vi "Create Fast Draw Object.vi"(6 "Actual Transform In":T1, 8 "error in (no error)":errorcluster, 9 "Multiplot Representation In":T3, 10 "3D Quiver.lvclass in":refnum<class "3D Quiver.lvclass">, 11 "Plot Object In":refnum<vi>) -> (0 "error out":errorcluster, 1 "Multiplot Representation Out":T3, 2 "3D Quiver.lvclass out":refnum<class "3D Quiver.lvclass">, 3 "Plot Object Out":refnum<vi>, 4 "Actual Transform Out":T1)   [LabVIEW 2020, in "3D Quiver.lvclass"]
uses:
  <vilib>/Math Plots/3D Math Plots/3D Quiver/3D Quiver/3D Quiver.lvclass
  <vilib>/Math Plots/3D Math Plots/3D Plot/3D Plot/Typedef/Multiplot Representation.ctl
  <vilib>/Math Plots/3D Math Plots/3D Plot/3D Plot/Typedef/Plot Representation.ctl
  <vilib>/Math Plots/3D Math Plots/3D Plot/3D Plot/Typedef/Range Clusters.ctl
  <vilib>/Math Plots/3D Math Plots/3D Plot/3D Plot/Typedef/Mesh Data.ctl
  <vilib>/Math Plots/3D Math Plots/3D Plot/3D Plot/Typedef/Actual Transform.ctl
  <vilib>/Math Plots/3D Math Plots/3D Quiver/3D Quiver/3D Quiver.lvclass/3D Quiver.ctl
  <vilib>/Math Plots/3D Math Plots/3D Plot/3D Plot/3D Plot.lvclass
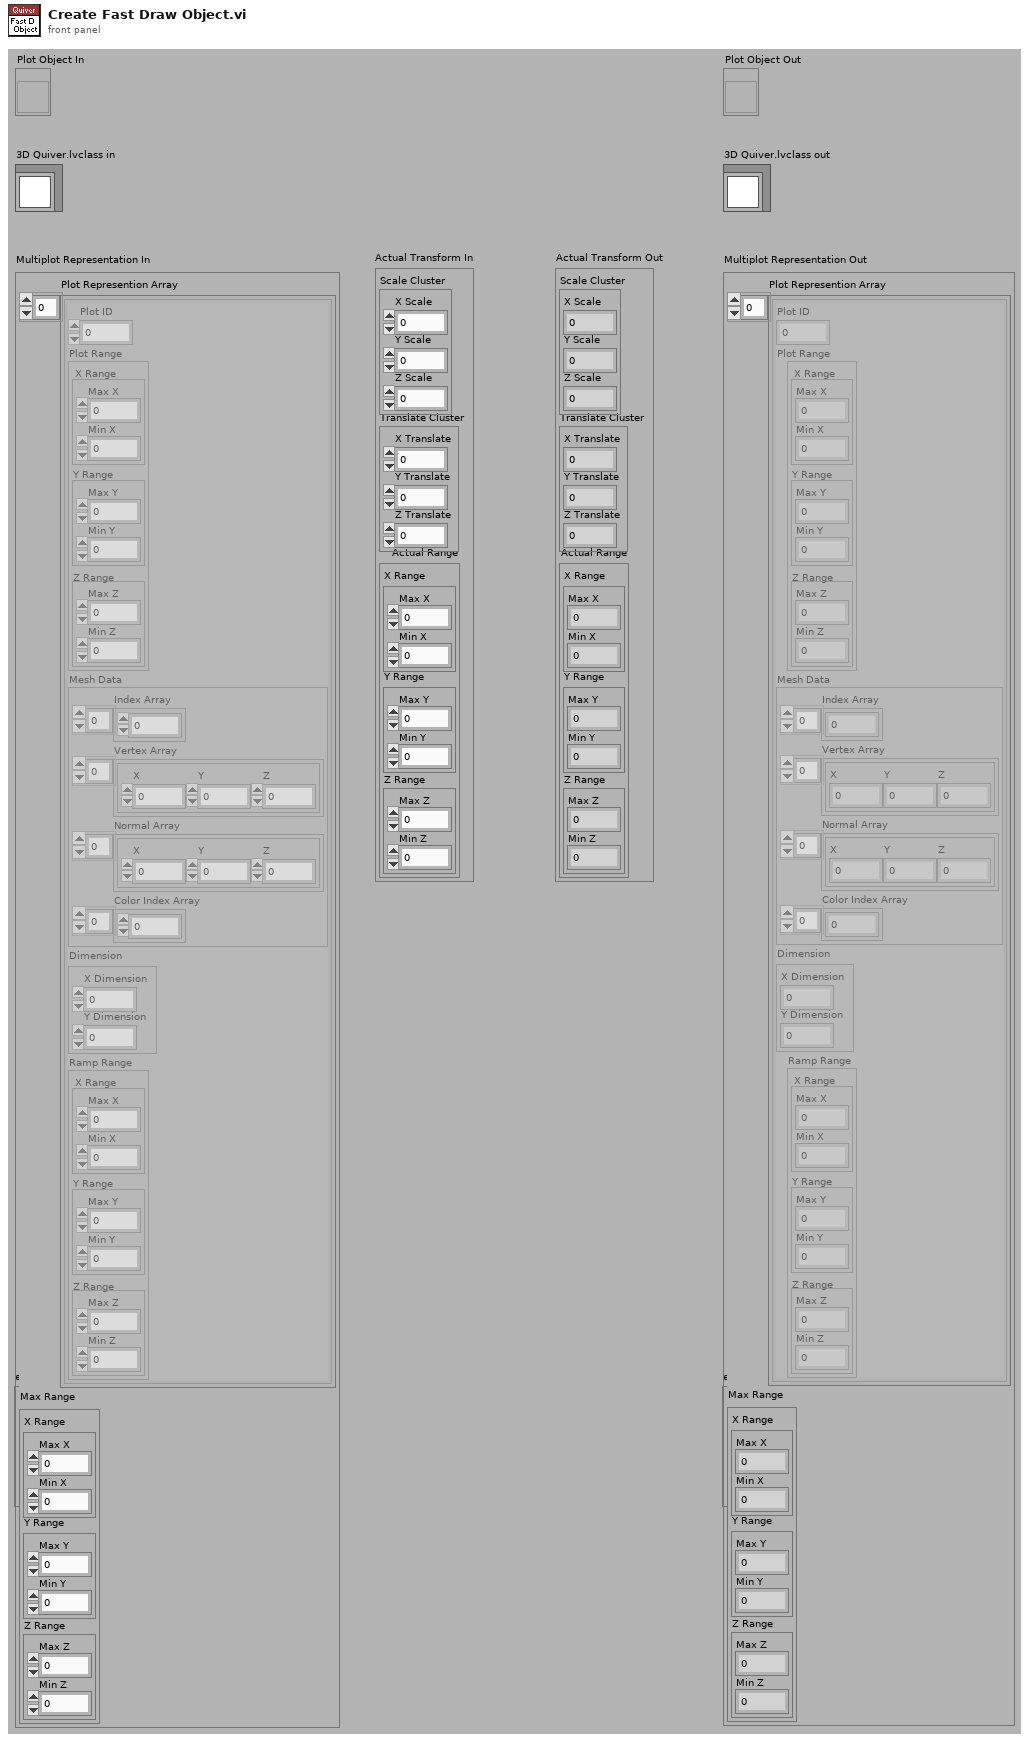
[diagram p1: front panel]
types:
  T1 = typedef "3D Plot.lvclass/Actual Transform.ctl" = cluster{"Scale Cluster":cluster{"X Scale":sgl, "Y Scale":sgl, "Z Scale":sgl}, "Translate Cluster":cluster{"X Translate":sgl, "Y Translate":sgl, "Z Translate":sgl}, "Actual Range":T2}
  T2 = typedef "3D Plot.lvclass/Range Clusters.ctl" = cluster{"X Range":cluster{"Max X":sgl, "Min X":sgl}, "Y Range":cluster{"Max Y":sgl, "Min Y":sgl}, "Z Range":cluster{"Max Z":sgl, "Min Z":sgl}}
  T3 = typedef "3D Plot.lvclass/Multiplot Representation.ctl" = cluster{"Plot Represention Array":T4[], "Max Range":T2}
  T4 = typedef "3D Plot.lvclass/Plot Representation.ctl" = cluster{"Plot ID":i32, "Plot Range":T2, "Mesh Data":T5, "Dimension":cluster{"X Dimension":i32, "Y Dimension":i32}, "Ramp Range":T2}
  T5 = typedef "3D Plot.lvclass/Mesh Data.ctl" = cluster{"Index Array":u32[], "Vertex Array":cluster{"X":sgl, "Y":sgl, "Z":sgl}[], "Normal Array":cluster{"X":sgl, "Y":sgl, "Z":sgl}[], "Color Index Array":i32[]}
  T6 = typedef "3D Quiver.lvclass/3D Quiver Property Array.ctl" = T7[]
  T7 = typedef "3D Quiver.lvclass/3D Quiver Property.ctl" = cluster{"General Property":cluster{"Plot Name":string, "Coordinate System":enum16{"Cartesian", "Cylindrical", "Spherical"}, "Opacity":sgl}, "Projection Property":cluster{"Draw XY":bool, "Draw YZ":bool, "Draw XZ":bool}, "Plot Property":cluster{"Line Style":T8, "Line Width":sgl, "Line Color":u32, "Antialiasing":bool, "Color Ramp Cluster":T9}, "Quiver Property":cluster{"Quvier Mode":enum16{"Quiver", "Quiver with surface"}, "Quiver Size":sgl, "Quiver Length":sgl}}
  T8 = typedef "3D Plot.lvclass/Line Type.ctl" = enum16{"None", "Solid", "Dash", "Dot", "Dash Dot"}
  T9 = typedef "3D Plot.lvclass/Color Ramp Cluster.ctl" = cluster{"Color Ramp Style":enum16{"None", "Shaded", "Color spectrum", "Grey scale", "Custom"}, "Color Ramp Array":u32[], "Color Ramp Index":i32[], "Interpolate?":bool, "Logarithm?":bool}
  T10 = enum16{"Points", "Lines", "Line Strip", "Line Loop", "Triangles", "Triangle Strip", "Triangle Fan", "Quads", "Quad Strip", "Polygon"}
  T11 = cluster{"Draw XY":bool, "Draw YZ":bool, "Draw XZ":bool}
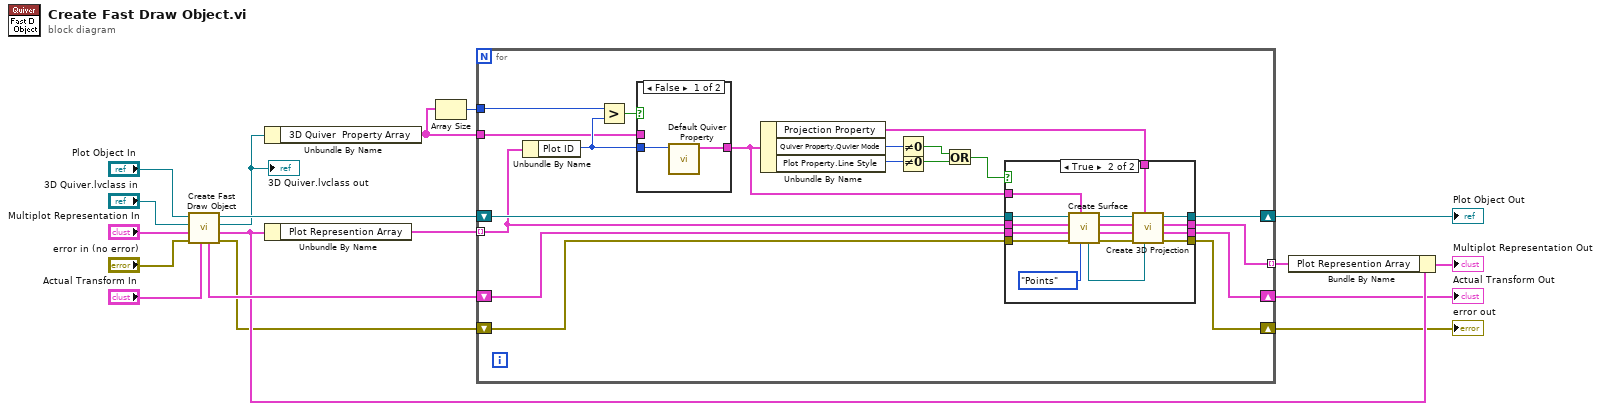
[diagram p0: block diagram]
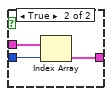
[diagram p2: hidden frame]
diagram:
  n1 = call-parent "Create Fast Draw Object.vi"("Actual Transform In"="Actual Transform In", "error in (no error)"="error in (no error)", "Multiplot Representation In"="Multiplot Representation In", "3D Plot.lvclass in"="3D Quiver.lvclass in", "Plot Object In"="Plot Object In") -> ("error out"=w3:errorcluster, "Multiplot Representation Out"=w9:T3, "3D Plot.lvclass out"=w4:refnum<class "3D Quiver.lvclass">, "Plot Object Out"=w11:refnum<vi>, "Actual Transform Out"=w10:T1)  [unwired: 2 out]
  "3D Quiver.lvclass out" <- w4
  n2 = Unbundle By Name(w4) -> ("3D Quiver  Property Array"=w2:T6)
  n3 = Unbundle By Name(w9) -> ("Plot Represention Array"=w13:T4[])
  n4 = Array Size(array=w2) -> (size(s)=w1:i32)
  n5 = for {
    tunnel: w2 -> [w20]
    tunnel: w13 -> [w33] mode=indexing
    tunnel: [w30] -> w12 mode=indexing
    shift-right: [w36] -> w6
    shift-left: w10 -> [w32]
    shift-right: [w35] -> w5
    shift-left: w3 -> [w31]
    shift-right: [w37] -> w7
    shift-left: w11 -> [w34]
    tunnel: w1 -> [w22]
    n6 = Unbundle By Name(w33) -> ("Plot ID"=w21:i32)
    n7 = Greater?(x=w22, y=w21) -> (0:w23:bool)
    n8 = case shown="False" w23 {
      tunnel: w20 -> [_ w42]
      tunnel: [w38 w41] -> w19
      tunnel: w21 -> [w39 w40]
      frame False {
        n9 = call <vilib>:"Default Quiver Property.vi"("Plot ID"=w39) -> ("Default Property"=w38:T7)  [unwired: 10 out]
      }
      frame True {
        n10 = Index Array(array=w42, index=w40) -> (element=w41:T7)
      }
    }
    n11 = Unbundle By Name(w19) -> ("Projection Property"=w29:T11, "Quiver Property.Quvier Mode"=w26:enum16{"Quiver", "Quiver with surface"}, "Plot Property.Line Style"=w25:T8)
    n12 = Not Equal To 0?(x=w26) -> (x != 0?=w28:bool)
    n13 = Not Equal To 0?(x=w25) -> (x != 0?=w27:bool)
    n14 = Or(x=w28, y=w27) -> (x .or. y?=w24:bool)
    n15 = case shown="True" w24 {
      tunnel: [w46 w61] -> w37
      tunnel: [w44 w60] -> w36
      tunnel: [w43 w59] -> w35
      tunnel: w34 -> [w46 w58]
      tunnel: w33 -> [w45 w57]
      tunnel: w32 -> [w44 w56]
      tunnel: w31 -> [w43 w55]
      tunnel: [w45 w51] -> w30
      tunnel: w29 -> [_ w49]
      tunnel: w19 -> [_ w47]
      frame False {
      }
      frame True {
        n16 = call <vilib>:"Create Surface.vi"("Draw Mode"=T10."Points", "3D Quvier Property"=w47, "error in (no error)"=w55, "Actual Transform In"=w56, "Plot Representation In"=w57, "Plot Object In"=w58) -> ("error out"=w53:errorcluster, "Actual Transform Out"=w52:T1, "Plot Representation Out"=w51:T4, "Plot Object Out"=w50:refnum<vi>, "Surface Object Out"=w54:refnum<vi>)  [unwired: 1 out]
        n17 = call <vilib>:"Create 3D Projection.vi"("Sub Object In"=w54, "Projection Property"=w49, "error in (no error)"=w53, "Actual Transform In"=w52, "Plot Object In"=w50) -> ("error out"=w59:errorcluster, "Actual Transform Out"=w60:T1, "Plot Object Out"=w61:refnum<vi>)  [unwired: 1 in, 3 out]
      }
    }
  }
  "error out" <- w5
  "Plot Object Out" <- w7
  "Actual Transform Out" <- w6
  n18 = Bundle By Name(cluster=w9, "Plot Represention Array"=w12) -> (→"Multiplot Representation Out":T3)
